vi "P_upd.vi"(2 "rho_max":dbl, 3 "P(t-1)":T1, 4 "error in (no error)":errorcluster, 5 "W_0":dbl, 6 "\\phi(t)":T1, 7 "\\Gamma(t)":T1) -> (0 "error out":errorcluster, 1 "P(t)":T1)   [LabVIEW 2021]
uses:
  <vilib>/Analysis/Matrix/Datatypes/RealMatrix.ctl
  <vilib>/Analysis/7linalg.llb/Eigenvalue and Vectors Output Option.ctl
  <vilib>/Analysis/Matrix/Numeric/Conversions/Array To Matrix - RA2.vi
  <vilib>/Analysis/Matrix/Numeric/Multiply/Multiply - RM,RM.vi
  <vilib>/Analysis/Matrix/Numeric/Multiply/Multiply - RM,R.vi
  <vilib>/Analysis/Matrix/Numeric/Subtract/Subtract - RM,RM.vi
  <vilib>/Analysis/7linalg.llb/Real Eigenvalues and Vectors.vi
  <vilib>/Analysis/Matrix/NI_Matrix.lvlib
  <vilib>/Analysis/NI_AALPro.lvlib
panel:
  out "max lambda(P(t))":dbl
  out "\\phi^T (t)":T1
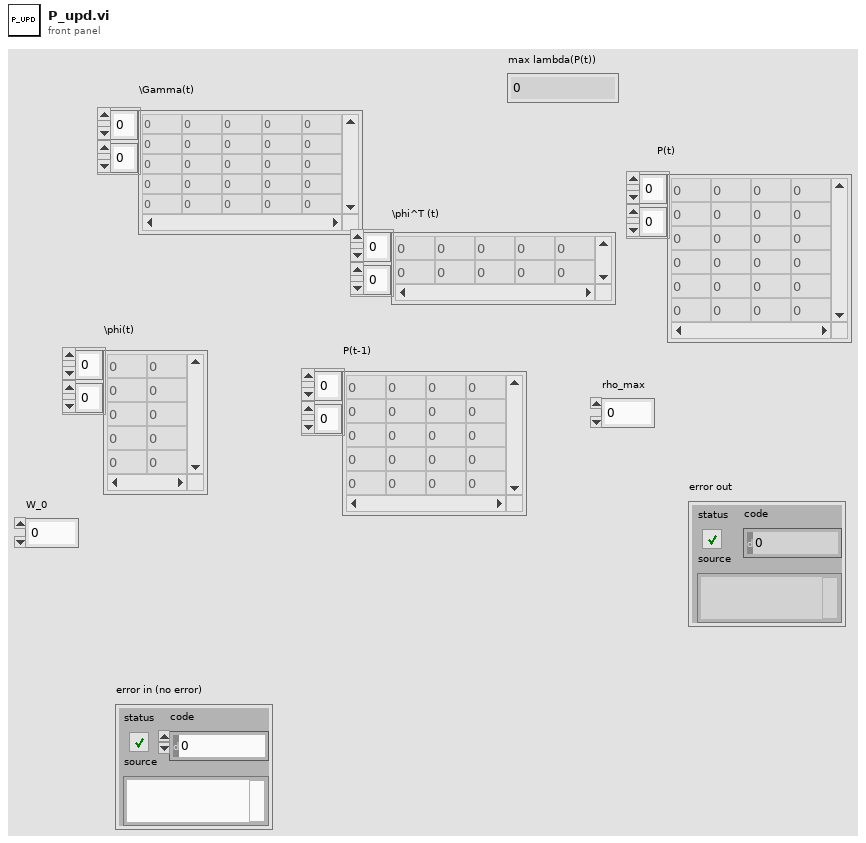
[diagram p1: front panel]
types:
  T1 = typedef "NI_Matrix.lvlib/RealMatrix.ctl" = dbl[][]
  T2 = typedef "NI_AALPro.lvlib/Eigenvalue and Vectors Output Option.ctl" = i32
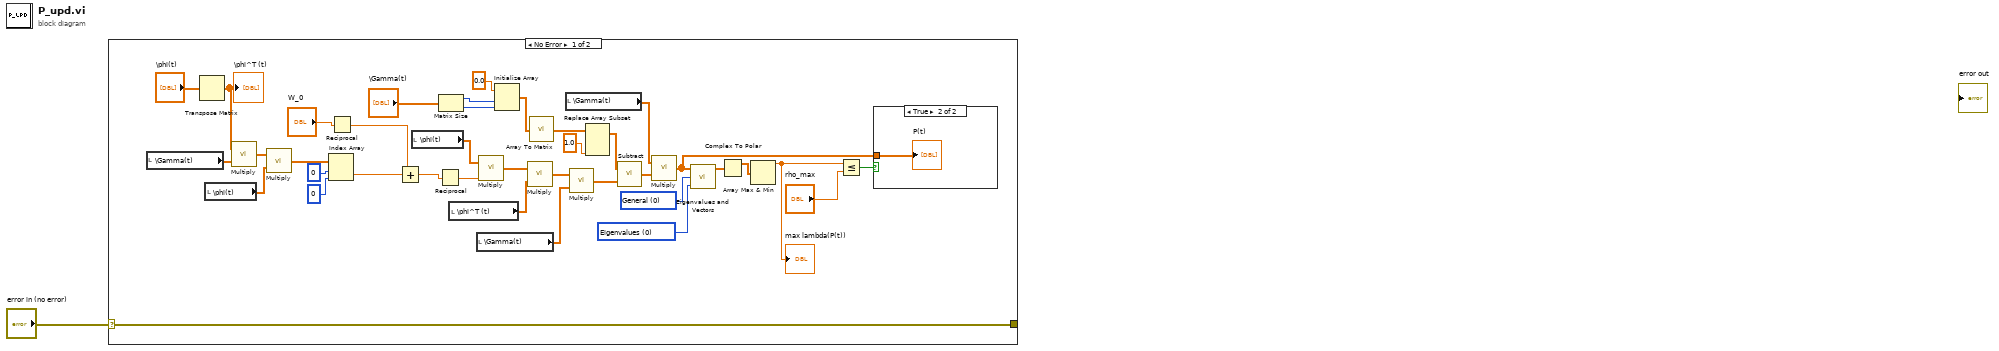
[diagram p0: block diagram]
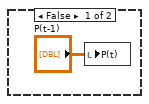
[diagram p2: hidden frame]
diagram:
  n1 = case shown="No Error" "error in (no error)" {
    selector: "error in (no error)" -> [w15 w42]
    tunnel: [w15 w42] -> _
    frame No Error {
      w13 = 0 items=["General", "Symmetric"] ("matrix type")
      w14 = T2 0 items=["Eigenvalues", "Eigenvalues & Vectors"] ("output option")
      n2 = local read "\\Gamma(t)"() -> (w31:T1)
      n3 = Transpose Matrix(1:"\\phi(t)") -> (0:w19:T1)
      "\\phi^T (t)" <- w19
      n4 = local read "\\phi(t)"() -> (w29:T1)
      n5 = call-poly <vilib>:"Multiply.vi"("Real Matrix B"=w31, "Real Matrix A"=w19) -> ("A * B"=w30:T1)
      n6 = call-poly <vilib>:"Multiply.vi"("Real Matrix B"=w29, "Real Matrix A"=w30) -> ("A * B"=w18:T1)
      n7 = Index Array(array=w18, index (row)=0, index (col)=0) -> (element=w4:dbl)
      n8 = Reciprocal(x="W_0") -> (1/x=w5:dbl)
      n9 = Add ("Add.vi")(x=w5, y=w4) -> (x+y=w3:dbl)
      n10 = local read "\\phi(t)"() -> (w28:T1)
      n11 = Reciprocal(x=w3) -> (1/x=w2:dbl)
      n12 = Matrix Size(0:"\\Gamma(t)") -> (1:w39:i32, 2:w38:i32)
      n13 = local read "\\phi^T (t)"() -> (w26:T1)
      n14 = local read "\\Gamma(t)"() -> (w21:T1)
      n15 = call-poly <vilib>:"Multiply.vi"("Real Scalar c"=w2, "Real Matrix A"=w28) -> ("A * c"=w27:T1)
      n16 = Initialize Array(0.0 ("element"), w39, w38) -> (w36:dbl[][])
      n17 = call-poly <vilib>:"Multiply.vi"("Real Matrix B"=w26, "Real Matrix A"=w27) -> ("A * B"=w25:T1)
      n18 = call-poly <vilib>:"Array To Matrix.vi"("Real 2D Array"=w36) -> ("Real Matrix"=w35:T1)
      n19 = local read "\\Gamma(t)"() -> (w20:T1)
      n20 = call-poly <vilib>:"Multiply.vi"("Real Matrix B"=w21, "Real Matrix A"=w25) -> ("A * B"=w24:T1)
      n21 = Replace Array Subset(array=w35, new element=1.0 ("new diagonal/fill element")) -> (w33:T1)  [unwired: 2 in]
      n22 = call-poly <vilib>:"Subtract.vi"("Real Matrix B"=w24, "Real Matrix A"=w33) -> ("A - B"=w23:T1)
      n23 = call-poly <vilib>:"Multiply.vi"("Real Matrix B"=w23, "Real Matrix A"=w20) -> ("A * B"=w7:T1)
      n24 = call-poly <vilib>:"Eigenvalues and Vectors.vi"("output option"=w14, "matrix type"=w13, "Input Matrix"=w7) -> ("Eigenvalues"=w12:cdb[])  [unwired: 2 out]
      n25 = Complex To Polar(r * e^(i*theta)=w12) -> (r=w11:dbl[])  [unwired: 1 out]
      n26 = Array Max & Min(array=w11) -> (max value=w10:dbl)  [unwired: 3 out]
      "max lambda(P(t))" <- w10
      n27 = Less Or Equal?(x=w10, y="rho_max") -> (x <= y?=w8:bool)
      n28 = case shown="True" w8 {
        tunnel: w7 -> [_ w41]
        frame False {
          n29 = local write "P(t)"("P(t-1)") -> ()
        }
        frame True {
          "P(t)" <- w41
        }
      }
    }
    frame Error {
    }
  }
